vi "Platform Format.vi"(8 "error in (no error)":errorcluster, 9 "Length (0)":u8, 10 "Type (0:ASCii)":u16(ring) items=["ASCii", "PACKed"], 11 "VISA resource name":refnum<visa-resource-name>) -> (0 "error out":errorcluster, 3 "VISA resource name out":refnum<visa-resource-name>)   [LabVIEW 2018, in "LTB-1.lvlib" / "3150.lvlib"]
doc: "Selects the data format and Length. The Length parameter is optional for all data format, its meaning is dependent on the data format selected. If PACKed type is selected, the data is transferred in a array. The ASCii-type data is automatically identified by its syntax. Therefore, in these cases, the FORMat subsystem is only necessary to determine the output format."
uses:
  3150.lvlib
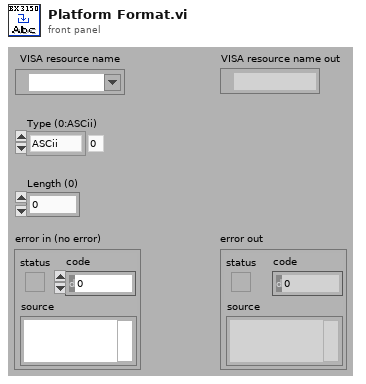
[diagram p1: front panel]
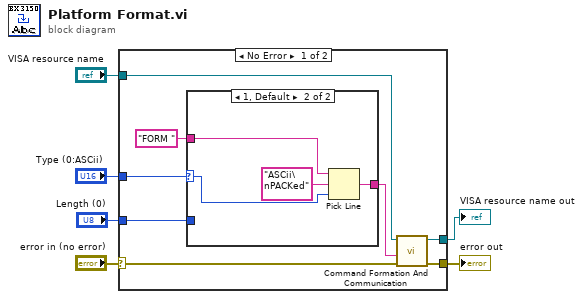
[diagram p0: block diagram]
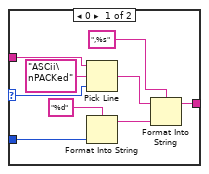
[diagram p2: hidden frame]
diagram:
  n1 = case shown="No Error" "error in (no error)" {
    selector: "error in (no error)" -> [w9 w29]
    tunnel: [w8 w28] -> w5
    tunnel: [w7 w29] -> w3
    tunnel: "VISA resource name" -> [w10 w28]
    tunnel: "Length (0)" -> [w13 _]
    tunnel: "Type (0:ASCii)" -> [w14 _]
    frame No Error {
      n2 = case shown="1, Default" w14 {
        selector: w14 -> [w20 w26]
        tunnel: w13 -> [w22 _]
        tunnel: "FORM " ("Command") -> [w19 w25]
        tunnel: [w15 w24] -> w11
        frame 0 {
          n3 = Pick Line(string ("")=w19, multi-line string="ASCii\nPACKed", line index=w20) -> (output string=w17:string)
          n4 = Format Into String(format string="%d", w22) -> (resulting string=w16:string)  [unwired: 2 in, 1 out]
          n5 = Format Into String(format string=",%s", initial string=w17, w16) -> (resulting string=w15:string)  [unwired: 1 in, 1 out]
        }
        frame 1, Default {
          n6 = Pick Line(string ("")=w25, multi-line string="ASCii\nPACKed", line index=w26) -> (output string=w24:string)
        }
      }
      n7 = call "Command Formation And Communication.vi"("error in (no error)"=w9, "Command"=w11, "VISA resource name"=w10) -> ("error out"=w7:errorcluster, "VISA resource name out"=w8:refnum<visa-resource-name>)  [unwired: 1 in, 6 out]
    }
    frame Error {
    }
  }
  "VISA resource name out" <- w5
  "error out" <- w3
